vi "Get Server Loop.vi"(8 "error in (no error)":errorcluster, 11 "TCP Server in":refnum<class "TCP Server.lvclass">) -> (0 "error out":errorcluster, 2 "Server Loop":bool, 3 "TCP Server out":refnum<class "TCP Server.lvclass">)   [LabVIEW 2012, in "Stream-TCP.lvlib" / "TCP Server.lvclass"]
uses:
  TCP Server.lvclass
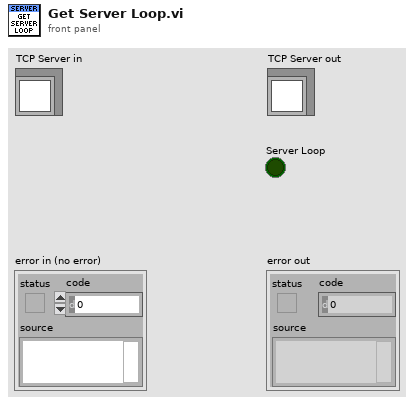
[diagram p1: front panel]
types:
  T1 = typedef "Stream-TCP.lvlib/TCP Server.lvclass/Ref Data.ctl" = cluster{"Listener":refnum<k5>, "Clients":refnum<class "TCP Client.lvclass">[], "Server Loop":bool}
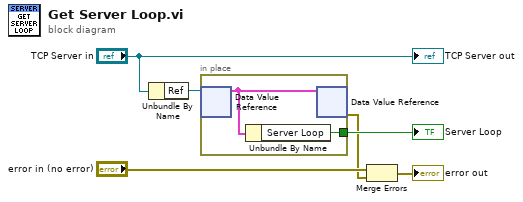
[diagram p0: block diagram]
diagram:
  n1 = Unbundle By Name("TCP Server in") -> ("Ref"=w5:refnum<data-value>)
  n2 = in-place {
    in-place-border: [w7] -> w3
    n3 = in-place-dvr #1(w5) -> (w8:T1)  [unwired: 1 out]
    n4 = Unbundle By Name(w8) -> ("Server Loop"=w7:bool)
    n5 = in-place-dvr #1(w8) -> (w1:errorcluster)  [unwired: 1 out]
  }
  "Server Loop" <- w3
  n6 = Merge Errors("error in (no error)", w1) -> (→"error out":errorcluster)
  "TCP Server out" <- "TCP Server in"
